vi "CONST820调试.vi"() -> ()   [LabVIEW 2017]
panel:
  out "VISA资源名称输出":refnum<visa-resource-name>
  in  "error in (no error) 2":errorcluster caption="错误输入（无错误）"
  in  "VISA resource name":refnum<visa-resource-name> caption="VISA资源名称"
  out "错误输出":errorcluster
  out "设定压力值":string
  in  "等待时间（毫秒）":u32=100
  in  "写":bool=TRUE
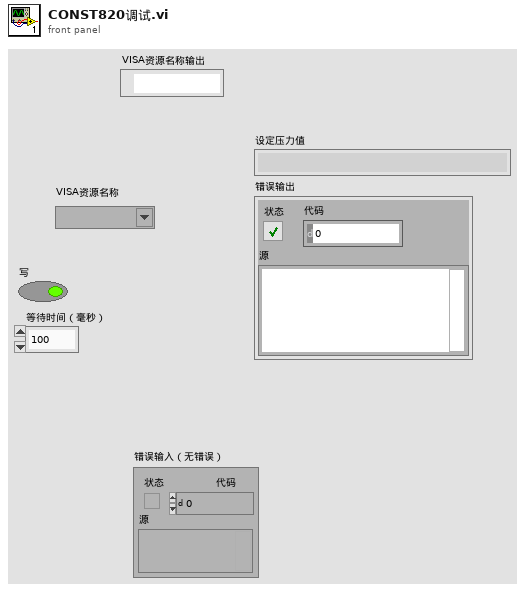
[diagram p1: front panel]
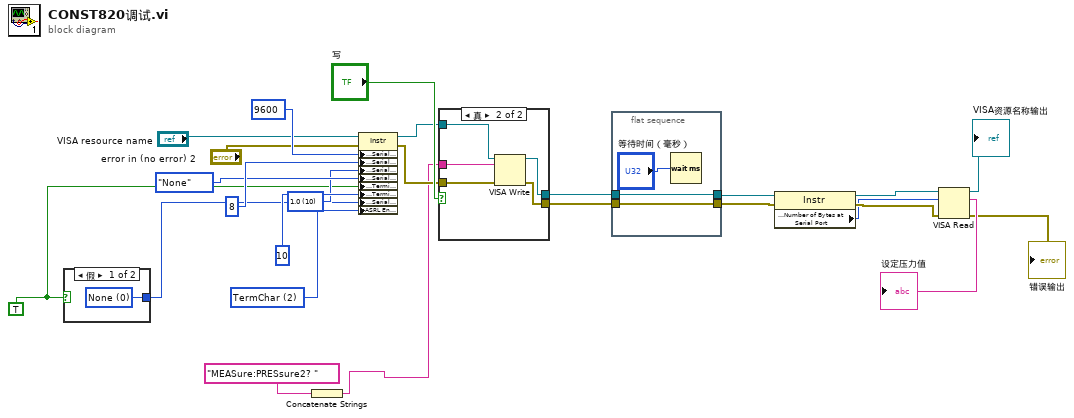
[diagram p0: block diagram]
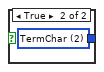
[diagram p2: hidden frame]
diagram:
  w8 = TRUE ("Enable Termination\nChar (T) 2")
  w7 = u16 2 items=["None", "Last Bit", "TermChar", "Break"] ("Serial Settings:End Mode for Writes")
  w10 = u16 10 items=["1.0"=10, "1.5"=15, "2.0"=20] ("stop bits (10: 1 bit)")
  n1 = case shown="假" w8 {
    tunnel: [w26 w27] -> w9
    frame False {
      w26 = u16 0 items=["None", "LastBit", "TermChar"] ("Serial Settings:Serial End Mode for Reads")
    }
    frame True {
      w27 = u16 2 items=["None", "LastBit", "TermChar"] ("Serial Settings:Serial End Mode for Reads")
    }
  }
  n2 = Concatenate Strings("MEASure:PRESsure2? ") -> (w1:string)
  n3 = property class="Instr"(reference="VISA resource name", error in="error in (no error) 2", "Serial Settings:Serial Baud Rate"=u32 9600 ("baud rate (9600)"), "Serial Settings:Serial Data Bits"=u16 8 ("data bits (8)"), "Serial Settings:Serial Stop Bits"=w10, "Serial Settings:Serial Parity"=enum16{"None", "Odd", "Even", "Mark", "Space"}."None" ("parity (0:none)"), "Message Based Settings:Termination Character Enable"=w8, "Message Based Settings:Termination Character"=u8 10 ("termination char\n(0xA = '\\n' = LF)"), "Serial Settings:Serial End Mode for Reads"=w9, "ASRL End Out"=w7) -> (reference out=w6:refnum<visa-resource-name>, error out=w5:errorcluster)
  n4 = case shown="真" "写" {
    tunnel: w1 -> [_ w34]
    tunnel: [w29 w33] -> w24
    tunnel: [w28 w32] -> w23
    tunnel: w6 -> [w28 w31]
    tunnel: w5 -> [w29 w30]
    frame False {
    }
    frame True {
      n5 = VISA Write(VISA resource name=w31, write buffer=w34, error in (no error)=w30) -> (VISA resource name out=w32:refnum<visa-resource-name>, error out=w33:errorcluster)  [unwired: 1 out]
    }
  }
  n6 = flat-sequence {
    tunnel: w24 -> [w35]
    tunnel: w23 -> [w36]
    tunnel: [w36] -> w20
    tunnel: [w35] -> w19
    frame #0 {
      n7 = Wait (ms)(milliseconds to wait="等待时间（毫秒）") -> ()  [unwired: 1 out]
    }
  }
  n8 = property class="Instr"(reference=w20, error in=w19) -> (reference out=w22:refnum<visa-resource-name>, error out=w21:errorcluster, "Serial Settings:Number of Bytes at Serial Port"=w18:u32)
  n9 = VISA Read(VISA resource name=w22, byte count=w18, error in (no error)=w21) -> (VISA resource name out=→"VISA资源名称输出":refnum<visa-resource-name>, read buffer=→"设定压力值":string, error out=→"错误输出":errorcluster)  [unwired: 1 out]
